vi "Write log.vi"(9 "text":string, 11 "log file":refnum<file>) -> (0 "status":bool, 2 "current time":timestamp format="%<%H:%M:%S%3u\n%Y/%m/%d>T")   [LabVIEW 2018]
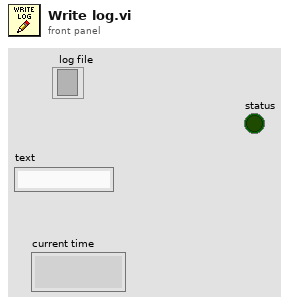
[diagram p1: front panel]
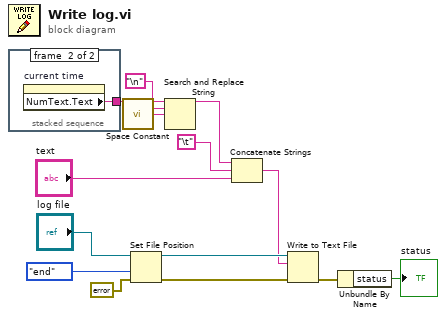
[diagram p0: block diagram]
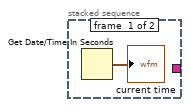
[diagram p2: hidden frame]
diagram:
  n1 = stacked-sequence {
    tunnel: [_ w16] -> w6
    frame #0 {
      n2 = Get Date/Time In Seconds() -> (seconds since 1Jan1904=→"current time":timestamp)
    }
    frame #1 {
      n3 = property on="current time" class="AbsTime (strict)"() -> ("NumText.Text"=w16:string)  [unwired: 2 in, 2 out]
    }
  }
  n4 = call <vilib>:"Space Constant.vi"() -> ("String"=w5:string)
  n5 = Set File Position(refnum="log file", from (0:start)=enum16{"start", "end", "current"}."end", error in=errorcluster {"status"=FALSE, "code"=0, "source"=""}) -> (refnum out=w11:refnum<file>, error out=w14:errorcluster)  [unwired: 1 in]
  n6 = Search and Replace String(input string=w6, search string="\n", replace string=w5) -> (result string=w3:string)  [unwired: 5 in, 3 out]
  n7 = Concatenate Strings(w3, "\t", "text") -> (w10:string)
  n8 = Write to Text File(file (use dialog)=w11, text=w10, error in=w14) -> (error out=w8:errorcluster)  [unwired: 1 in, 2 out]
  n9 = Unbundle By Name(w8) -> ("status"=→"status":bool)
